vi "initFirmware.vi"(8 "error in (no error)":errorcluster, 10 "TypeFirmware":T1, 11 "XuLyStringUART in":refnum<class "XuLyStringUART.lvclass">) -> (0 "error out":errorcluster, 3 "XuLyStringUART out":refnum<class "XuLyStringUART.lvclass">)   [LabVIEW 2017, in "LibraryGcode.lvlib" / "XuLyStringUART.lvclass"]
uses:
  XuLyStringUART.lvclass
  control/TypeFirmwareControl.ctl
  XuLyStringUART.lvclass/XuLyStringUART.ctl
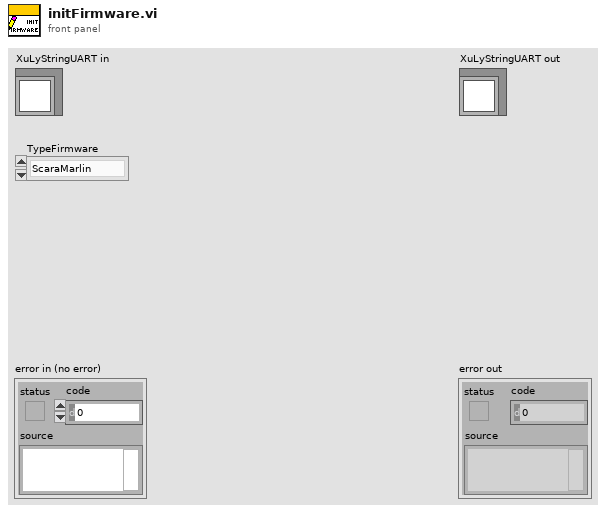
[diagram p1: front panel]
types:
  T1 = typedef "TypeFirmwareControl.ctl" = enum16{"ScaraMarlin", "CncMarlin", "Mk4Due"}
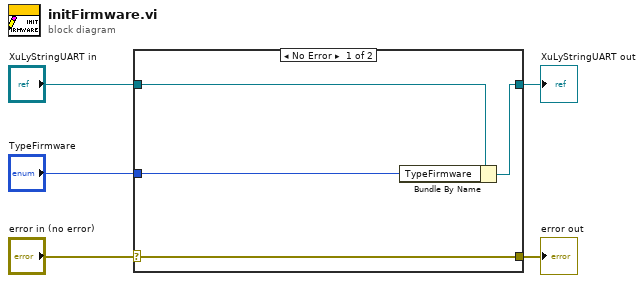
[diagram p0: block diagram]
diagram:
  n1 = case shown="No Error" "error in (no error)" {
    selector: "error in (no error)" -> [w9 w10]
    tunnel: [w9 w10] -> w4
    tunnel: [w7 w11] -> w2
    tunnel: "XuLyStringUART in" -> [w8 w11]
    tunnel: "TypeFirmware" -> [w6 _]
    frame No Error {
      n2 = Bundle By Name(cluster=w8, "TypeFirmware"=w6) -> (w7:refnum<class "XuLyStringUART.lvclass">)
    }
    frame Error {
    }
  }
  "error out" <- w4
  "XuLyStringUART out" <- w2
